vi "Output Motor Enable Bits.vi"   [LabVIEW 2010]
uses:
  <vilib>/eio/EIONode/EIONode.xnode
  Motor Encoder Global.vi
  Motor Output Global.vi
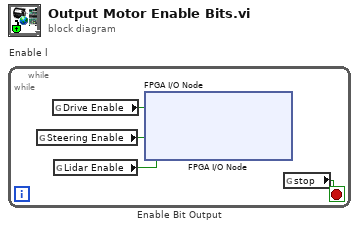
[diagram p0: block diagram]
diagram:
  n1 = while "Enable l" {
    stop <- w4 stop-if-true
    n2 = global read "Motor Output Global.vi" "Steering Enable"() -> (w2:bool)
    n3 = global read "Motor Output Global.vi" "Drive Enable"() -> (w3:bool)
    n4 = global read "Motor Output Global.vi" "Lidar Enable"() -> (w1:bool)
    n5 = xnode "FPGA I/O Node"("Drive Motor Enable"=w3, "Steering Motor Inhibit"=w2, "Lidar Motor Inhibit"=w1) -> ()  [unwired: 3 in, 3 out]
    n6 = global read "Motor Encoder Global.vi" "stop"() -> (w4:bool)
  }
  n7 = while "Enable Bit Output" {
    stop <- w8 stop-if-true
    n8 = global read "Motor Output Global.vi" "Steering Enable"() -> (w6:bool)
    n9 = global read "Motor Output Global.vi" "Drive Enable"() -> (w7:bool)
    n10 = global read "Motor Output Global.vi" "Lidar Enable"() -> (w5:bool)
    n11 = xnode "FPGA I/O Node"("Drive Motor Enable"=w7, "Steering Motor Inhibit"=w6, "Lidar Motor Inhibit"=w5) -> ()  [unwired: 3 in, 3 out]
    n12 = global read "Motor Encoder Global.vi" "stop"() -> (w8:bool)
  }
